vi "Create Test Suite (Template).vi"(5 "Interactive (T)":bool=TRUE, 7 "Verbose (F)":bool, 8 "error in (no error)":errorcluster, 9 "Test Report":refnum<class "Test Report.lvclass">, 11 "Test Runner.Template in":refnum<class "caraya unit tests.lvclass">) -> (0 "error out":errorcluster, 3 "Test Runner.Template out":refnum<class "caraya unit tests.lvclass">)   [LabVIEW 2023, in "caraya unit tests.lvclass"]
uses:
  caraya unit tests.lvclass
  <vilib>/addons/_JKI Toolkits/Caraya/classes/Test Report/Test Report.lvclass
  <vilib>/addons/_JKI Toolkits/Caraya/classes/Test Runner/Test Runner.lvclass/Test Runner.ctl
  caraya unit tests.lvclass/caraya unit tests.ctl
  <vilib>/addons/_JKI Toolkits/Caraya/classes/Test Runner/Test Runner.lvclass
  C:/Program Files/National Instruments/LabVIEW 2023/vi.lib/addons/_JKI Toolkits/Caraya/classes/Test Runner/Test Runner.lvclass
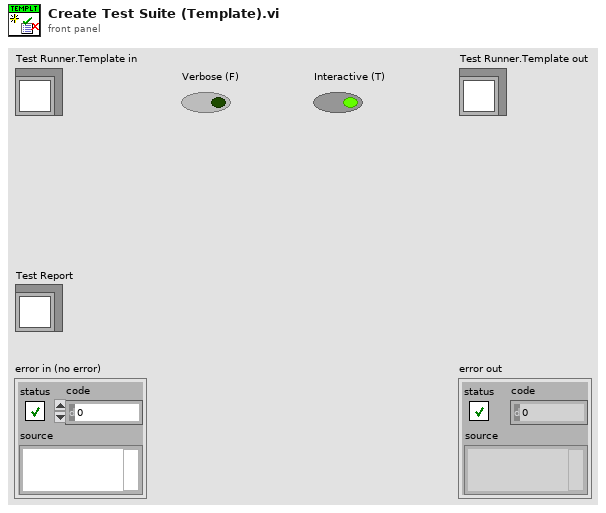
[diagram p1: front panel]
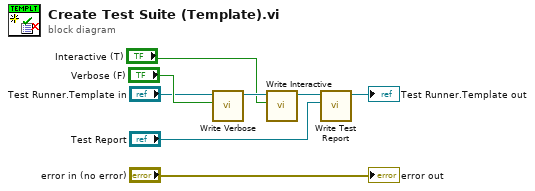
[diagram p0: block diagram]
diagram:
  n1 = call <vilib>:"Write Verbose.vi"("Verbose"="Verbose (F)", "Test Runner in"="Test Runner.Template in") -> ("Test Runner out"=w6:refnum<class "caraya unit tests.lvclass">)  [unwired: 9 in]
  n2 = call <vilib>:"Write Interactive.vi"("Interactive"="Interactive (T)", "Test Runner in"=w6) -> ("Test Runner out"=w3:refnum<class "caraya unit tests.lvclass">)  [unwired: 9 in]
  n3 = call <vilib>:"Write Test Report.vi"("Test Report"="Test Report", "Test Runner in"=w3) -> ("Test Runner in"=→"Test Runner.Template out":refnum<class "caraya unit tests.lvclass">)  [unwired: 9 in]
  "error out" <- "error in (no error)"
